vi "Spartan Builder - Build Database.vi"(8 "error in":errorcluster, 11 "Database Version":T1 {"Build Date/Time" format="%<%X\n%x>T"}) -> (0 "error out":errorcluster)   [LabVIEW 2011]
doc: "Use this VI Template to create a custom Pre-/Post-Build VI."
uses:
  server/database/Fields/Field System Fields.ctl
  www/tests/Test Status.ctl
  SI.LIB/OGAB Version.ctl
  server/database/Fields/Field Order By.ctl
  server/database/Users/User Record.ctl
  server/database/History/History Record.ctl
  server/database/Fields/Field Record.ctl
  server/database/Fields/Field DataTypes.ctl
  server/database/Fields/Field NextItem.ctl
  <userlib>/_OpenG.lib/file/file.llb/Convert File Extension (Path)__ogtk.vi
panel:
  in  "Test Status":T2
  in  "System Fields":T3=enum."Serial_Number"
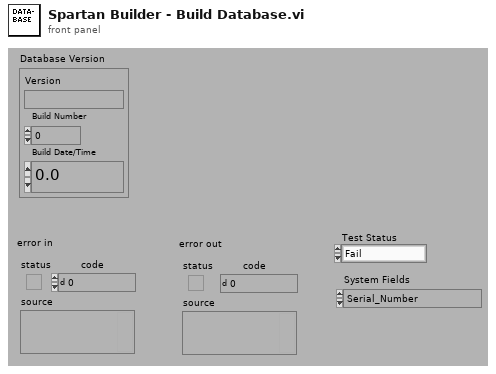
[diagram p1: front panel]
types:
  T1 = typedef "OGAB Version.ctl" = cluster{"Version":string, "Build Number":u32, "Build Date/Time":dbl}
  T2 = typedef "Test Status.ctl" = enum16{"Fail", "Pass", "Abort", "Error", "Done", "Pass by Sample", "Fail by Sample", "Pass Override", "Fail Override", "Not Tested"}
  T3 = typedef "Field System Fields.ctl" = enum32{"Company", "End_Timestamp", "Model_Number", "Operator", "Serial_Number", "Start_Timestamp", "Step_Number", "Step_Tag", "Test_Run", "Test_Sequence", "Test_Station", "Test_Station_Name", "Test_Status", "Test_Type", "Test_Version", "Spartan_Version_Created", "Spartan_Version_Current"}
  T4 = typedef "History Record.ctl" = cluster{"ixHistory":i32, "sVersion":string, "tUpdate":timestamp}
  T5 = typedef "User Record.ctl" = cluster{"ixUser":i32, "sxUsername":string, "sLastName":string, "sFirstName":string, "sEmail":string, "sPassword":string, "tLoginTime":timestamp, "sLoginComputer":string, "fAdministrator":bool, "fRunSequences":bool, "fModifySequences":bool, "fRunScenarios":bool, "fModifyScenarios":bool, "fModifyTemplates":bool, "fModifyUsers":bool, "fModifyStations":bool, "fModifyFields":bool}
  T6 = typedef "Field Order By.ctl" = enum32{"sxSequenceId", "sxFieldId", "sDisplayName", "sValue", "fSetAtTest", "fRequired", "nNextItem"}
  T7 = typedef "Connection Refnum.ctl" = cluster{"Environment Handle":i32, "Connection Handle":i32}
  T8 = typedef "Field Record.ctl" = cluster{"ixField":i32, "iSequenceOrder":i32, "sxFieldId":string, "sxSequenceId":string, "sDisplayName":string, "sValue":string, "sUnits":string, "nDataType":T9, "nNextItem":T10, "fSystem":bool, "fSystemValue":bool, "fRequired":bool, "fSetAtTest":bool, "fTestField":bool, "fDeleted":bool, "fIndexed":bool, "fFreeList":bool}
  T9 = typedef "Field DataTypes.ctl" = enum32{"text", "numeric", "list", "timestamp", "boolean"}
  T10 = typedef "Field NextItem.ctl" = enum32{"Reset", "Retain", "Auto-Increment"}
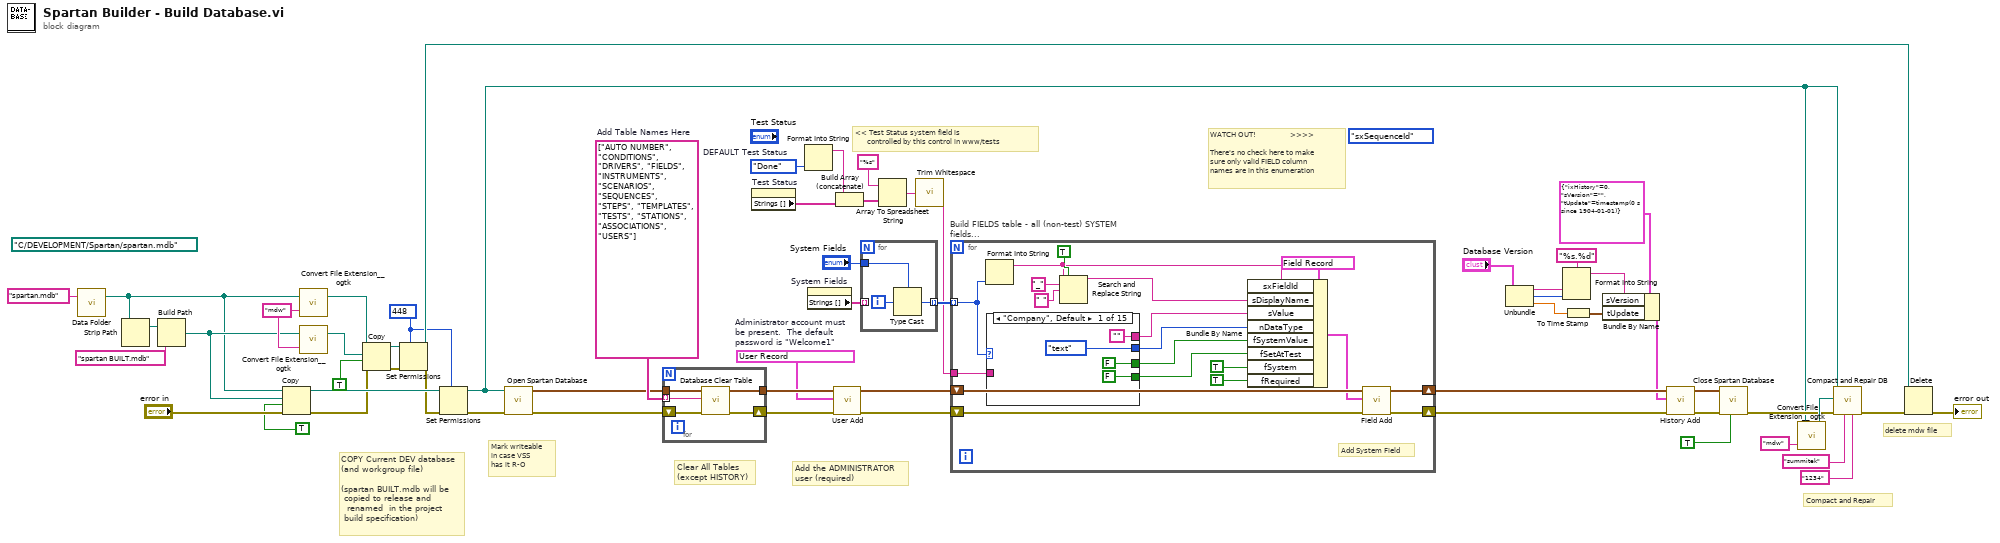
[diagram p0: block diagram]
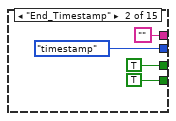
[diagram p2: hidden frame]
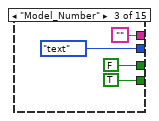
[diagram p3: hidden frame]
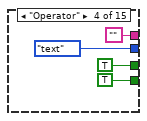
[diagram p4: hidden frame]
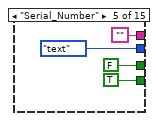
[diagram p5: hidden frame]
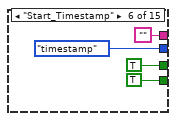
[diagram p6: hidden frame]
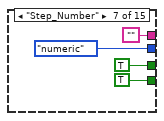
[diagram p7: hidden frame]
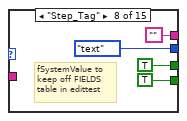
[diagram p8: hidden frame]
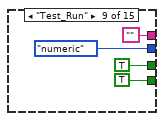
[diagram p9: hidden frame]
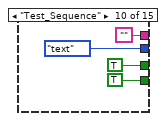
[diagram p10: hidden frame]
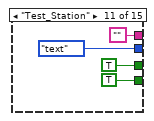
[diagram p11: hidden frame]
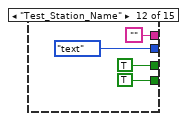
[diagram p12: hidden frame]
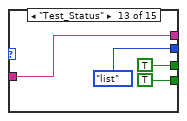
[diagram p13: hidden frame]
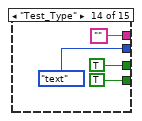
[diagram p14: hidden frame]
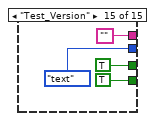
[diagram p15: hidden frame]
diagram:
  w5 = i16 448 ("permissions")
  w16 = "mdw" ("new ending (none)")
  (unwired) path "C:/DEVELOPMENT/Spartan/spartan.mdb" ("appended path")
  w41 = Test_Status."Done"  # DEFAULT Test Status
  w49 = T5 {"ixUser"=1, "sxUsername"="Administrator", "sLastName"="Administrator", "sFirstName"="Administrator", "sEmail"="", "sPassword"="D318F44739DCED66793B1A603028133A76AE680E", "tLoginTime"=timestamp(0 s since 1904-01-01), "sLoginComputer"="", "fAdministrator"=TRUE, "fRunSequences"=TRUE, "fModifySequences"=TRUE, "fRunScenarios"=TRUE, "fModifyScenarios"=TRUE, "fModifyTemplates"=TRUE, "fModifyUsers"=TRUE, "fModifyStations"=TRUE, "fModifyFields"=TRUE}  # Administrator account must be present.  The default password is "Welcome1"
  (unwired) Field_Order_By."sxSequenceId" ("Fields Order By")
  w58 = string[] ["AUTO NUMBER", "CONDITIONS", "DRIVERS", "FIELDS", "INSTRUMENTS", "SCENARIOS", "SEQUENCES", "STEPS", "TEMPLATES", "TESTS", "STATIONS", "ASSOCIATIONS", "USERS"]  # Add Table Names Here
  # "delete mdw file"
  # "Compact and Repair"
  # "<< Test Status system field is\n      controlled by this control in www/tests"
  # "Add the ADMINISTRATOR\nuser (required)"
  # "WATCH OUT!                 >>>>\n\nThere's no check here to make\nsure only valid FIELD column\nnames are in this enumeration"
  # "Mark writeable\nin case VSS\nhas it R-O"
  # "COPY Current DEV database\n(and workgroup file)\n\n(spartan BUILT.mdb will be\n copied to release and\n  renamed  in the project\n build specification)"
  # "Clear All Tables\n(except HISTORY)"
  n1 = call "Data Folder.vi"("Relative Path (\"\" - Folder)"="spartan.mdb" ("Relative Path (\"\" - Folder)")) -> ("Data Folder"=w2:path)  [unwired: 2 in]
  n2 = Strip Path(path=w2) -> (stripped path=w56:path)  [unwired: 1 out]
  n3 = Build Path(base path=w56, name or relative path="spartan BUILT.mdb") -> (appended path=w13:path)
  n4 = Copy(8:"error in", 9:TRUE, 10:w13, 11:w2) -> (0:w17:errorcluster, 3:w19:path)  [unwired: 2 out]
  n5 = call-poly <userlib>:"Convert File Extension__ogtk.vi"("new ending (none)"=w16, "file name"=w2) -> ("new filename"=w15:path)  [unwired: 1 out]
  n6 = call-poly <userlib>:"Convert File Extension__ogtk.vi"("new ending (none)"=w16, "file name"=w13) -> ("new filename"=w14:path)  [unwired: 1 out]
  n7 = Copy(8:w17, 9:TRUE, 10:w14, 11:w15) -> (0:w6:errorcluster, 3:w9:path)  [unwired: 2 out]
  n8 = Set Permissions(7:w5, 8:w6, 11:w9) -> (0:w7:errorcluster, 3:w8:path)  [unwired: 2 out]
  n9 = Set Permissions(7:w5, 8:w7, 11:w19) -> (0:w55:errorcluster, 3:w4:path)  [unwired: 2 out]
  n10 = call "Open Spartan Database.vi"("error in (no error)"=w55, "DB Path (empty - use default)"=w4) -> ("error out"=w12:errorcluster, "Connection Refnum"=w54:T7)  [unwired: 1 in, 7 out]
  n11 = for {
    shift-right: [w63] -> w51
    shift-left: w12 -> [w64]
    tunnel: w54 -> [w62]
    tunnel: [w61] -> w52
    tunnel: w58 -> [w60] mode=indexing
    n12 = call "Database Clear Table.vi"("error in (no error)"=w64, "Table Name (\"\")"=w60, "Connection Refnum"=w62) -> ("error out"=w63:errorcluster, "Connection Refnum"=w61:T7)  [unwired: 7 out]
  }
  n13 = property on="Test Status" class="Enum (strict)"() -> ("Strings []"=w40:string[])  [unwired: 2 in, 2 out]
  n14 = Format Into String(w41) -> (resulting string=w42:string)  [unwired: 3 in, 1 out]
  n15 = property on="System Fields" class="Enum (strict)"() -> ("Strings []"=w48:string[])  [unwired: 2 in, 2 out]
  n16 = call "User Add.vi"("error in (no error)"=w51, "User Record"=w49, "Connection Refnum"=w52) -> ("error out"=w50:errorcluster, "Connection Refnum"=w53:T7)  [unwired: 7 out]
  n17 = Build Array (concatenate)(w42, w40) -> (w43:string[])
  n18 = for {
    tunnel: "System Fields" -> [w66]
    tunnel: [w65] -> w46 mode=indexing
    tunnel: w48 -> [_] mode=indexing
    i -> [w67]
    n19 = Type Cast(type=w66, x=w67) -> (*(type *) &x=w65:T3)
  }
  n20 = Array To Spreadsheet String(array=w43, 3:"%s") -> (spreadsheet string=w45:string)  [unwired: 1 out]
  n21 = call <vilib>:"Trim Whitespace.vi"("string"=w45) -> ("trimmed string"=w39:string)  [unwired: 1 in]
  n22 = for "Build FIELDS table - all (non-test) SYSTEM fields..." {
    shift-right: [w83] -> w27
    shift-left: w53 -> [w85]
    shift-right: [w84] -> w29
    shift-left: w50 -> [w86]
    tunnel: w46 -> [w73] mode=indexing
    tunnel: w39 -> [w68]
    # "Add System Field"
    n23 = Format Into String(w73) -> (resulting string=w74:string)  [unwired: 3 in, 1 out]
    n24 = case shown="\"Company\", Default" w73 {
      tunnel: ["" "" "" "" "" "" "" "" "" "" "" "" w135 "" ""] -> w72
      tunnel: [Field_DataTypes."text" ("nDataType") Field_DataTypes."timestamp" ("nDataType") Field_DataTypes."text" ("nDataType") Field_DataTypes."text" ("nDataType") Field_DataTypes."text" ("nDataType") Field_DataTypes."timestamp" ("nDataType") Field_DataTypes."numeric" ("nDataType") Field_DataTypes."text" ("nDataType") Field_DataTypes."numeric" ("nDataType") Field_DataTypes."text" ("nDataType") Field_DataTypes."text" ("nDataType") Field_DataTypes."text" ("nDataType") Field_DataTypes."list" ("nDataType") Field_DataTypes."text" ("nDataType") Field_DataTypes."text" ("nDataType")] -> w71
      tunnel: [FALSE TRUE FALSE TRUE FALSE TRUE TRUE TRUE TRUE TRUE TRUE TRUE TRUE TRUE TRUE] -> w70
      tunnel: [FALSE TRUE TRUE TRUE TRUE TRUE TRUE TRUE TRUE TRUE TRUE TRUE TRUE TRUE TRUE] -> w69
      tunnel: w68 -> [_ _ _ _ _ _ _ _ _ _ _ _ w135 _ _]
      frame "Company", Default {
      }
      frame "End_Timestamp" {
      }
      frame "Model_Number" {
      }
      frame "Operator" {
      }
      frame "Serial_Number" {
      }
      frame "Start_Timestamp" {
      }
      frame "Step_Number" {
      }
      frame "Step_Tag" {
        # "fSystemValue to\nkeep off FIELDS\ntable in edittest"
      }
      frame "Test_Run" {
      }
      frame "Test_Sequence" {
      }
      frame "Test_Station" {
      }
      frame "Test_Station_Name" {
      }
      frame "Test_Status" {
      }
      frame "Test_Type" {
      }
      frame "Test_Version" {
      }
    }
    n25 = Search and Replace String(replace all?=TRUE, input string=w74, search string="_", replace string=" ") -> (result string=w77:string)  [unwired: 1 in, 6 out]
    n26 = Bundle By Name(cluster=T8 {"ixField"=0, "iSequenceOrder"=0, "sxFieldId"="", "sxSequenceId"="", "sDisplayName"="", "sValue"="", "sUnits"="", "nDataType"=enum."timestamp", "nNextItem"=enum."Reset", "fSystem"=FALSE, "fSystemValue"=FALSE, "fRequired"=FALSE, "fSetAtTest"=FALSE, "fTestField"=FALSE, "fDeleted"=FALSE, "fIndexed"=FALSE, "fFreeList"=FALSE} ("Field Record"), "sxFieldId"=w74, "sDisplayName"=w77, "sValue"=w72, "nDataType"=w71, "fSystemValue"=w70, "fSetAtTest"=w69, "fSystem"=TRUE, "fRequired"=TRUE) -> (w81:T8)
    n27 = call "Field Add.vi"("error in (no error)"=w86, "Field Record"=w81, "Connection Refnum"=w85) -> ("error out"=w84:errorcluster, "Connection Refnum"=w83:T7)  [unwired: 1 in, 6 out]
  }
  n28 = Unbundle("Database Version") -> ("Version"=w23:string, "Build Number"=w22:u32, "Build Date/Time"=w21:dbl)
  n29 = Format Into String(format string="%s.%d", w23, w22) -> (resulting string=w32:string)  [unwired: 2 in, 1 out]
  n30 = To Time Stamp(1:w21) -> (0:w33:timestamp)
  n31 = Bundle By Name(cluster=T4 {"ixHistory"=0, "sVersion"="", "tUpdate"=timestamp(0 s since 1904-01-01)} ("History Record"), "sVersion"=w32, "tUpdate"=w33) -> (w25:T4)
  n32 = call "History Add.vi"("error in (no error)"=w29, "History Record"=w25, "Connection Refnum"=w27) -> ("error out"=w28:errorcluster, "Connection Refnum"=w26:T7)  [unwired: 7 out]
  n33 = call "Close Spartan Database.vi"("Force Close? (f)"=TRUE, "error in (no error)"=w28, "Connection Refnum"=w26) -> ("error out"=w35:errorcluster)  [unwired: 2 in, 6 out]
  n34 = call-poly <userlib>:"Convert File Extension__ogtk.vi"("new ending (none)"="mdw", "file name"=w4) -> ("new filename"=w37:path)  [unwired: 1 out]
  n35 = call "Compact and Repair DB.vi"("password (\"\")"="1234" ("password (\"\")"), "username (\"\")"="summitek" ("username (\"\")"), "error in (no error)"=w35, "Workgroup DB (none)"=w37, "Database Path (empty)"=w4) -> ("error out"=w11:errorcluster)  [unwired: 6 out]
  n36 = Delete(path (use dialog)=w8, error in=w11) -> (error out=→"error out":errorcluster)  [unwired: 5 out]
